vi "STC31-string-array-to-data.vi"(9 "Starting Index":i32, 11 "Data In (string array)":string[](array[string])) -> (2 "STC31: Temp (degC)":dbl format="%.2f", 3 "STC31: CO2 (ppm)":dbl format="%.2f")   [LabVIEW 2021]
panel:
  out "STC31: Temp":string
  out "STC31: CO2":string
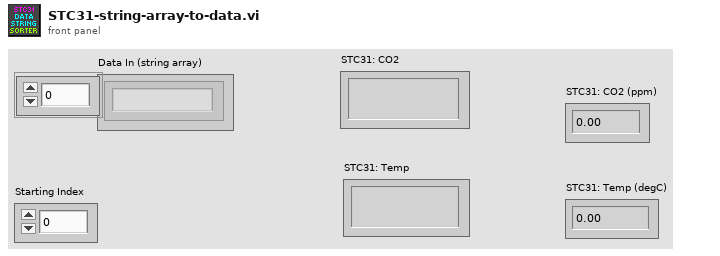
[diagram p1: front panel]
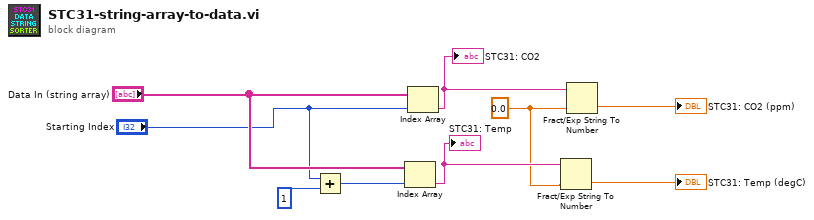
[diagram p0: block diagram]
diagram:
  w2 = 0.0
  n1 = Add(x="Starting Index", y=1) -> (x+y=w7:i32)
  n2 = Index Array(array="Data In (string array)", index=w7) -> (element=w3:string)
  "STC31: Temp" <- w3
  n3 = Index Array "Index Array"(array="Data In (string array)", index="Starting Index") -> (element=w5:string)
  "STC31: CO2" <- w5
  n4 = Fract/Exp String To Number(string=w3, default (0 dbl)=w2) -> (number=→"STC31: Temp (degC)":dbl)  [unwired: 2 in, 1 out]
  n5 = Fract/Exp String To Number(string=w5, default (0 dbl)=w2) -> (number=→"STC31: CO2 (ppm)":dbl)  [unwired: 2 in, 1 out]
